vi "Add Subscriber.vi"(8 "error in (no error)":errorcluster, 10 "New FIFO Instance Config":T2 {"Custom Data" format="%.0x"}, 11 "CIF_CIPC_Chn in":refnum<class "CIF_CIPC_Chn.lvclass">) -> (0 "error out":errorcluster, 2 "New FIFO Instance":T1 {"Custom Data" format="%.0x"}, 3 "CIF_CIPC_Chn out":refnum<class "CIF_CIPC_Chn.lvclass">)   [LabVIEW 2021, in "CIF_CIPC_Chn.lvclass"]
uses:
  CIF_CIPC_Chn.lvclass
  D:/dev/Packages/CIF_Channels_Core/src/CIFChannels/CIFChannels.lvclass
  ChannelCommon/typedef/New FIFO Instance Configuration.ctl
  ChannelCommon/typedef/New FIFO Instance Response.ctl
  CIFChannels/CIFChannels.lvclass/CIFChannels.ctl
  CIF_CIPC_Chn.lvclass/CIF_CIPC_Chn.ctl
  ChannelCommon/typedef/Errors.ctl
  CIFChannels/Accessors/Read Name.vi
  <vilib>/CIF Foundation/CIF Utilities/Errors/Append Error Location.vi
  SubVIs/Flatten Buffer Configuration.vi
  <vilib>/CIF Foundation/CIF CIPC/Utilities/Get Size.vi
  ChannelCommon/Utilities/Unflatten FIFO Config.vi
  ChannelCommon/Utilities/Flatten FIFO Config.vi
  CIFChannels/Accessors/Read Channel State.vi
  CIFChannels/Accessors/Read Custom Config Data.vi
  <vilib>/CIF Foundation/CIF Utilities/DataTypes/Flatten Unflatten/Flatten U32.vi
  <vilib>/CIF Foundation/CIF Utilities/DataTypes/Flatten Unflatten/Flatten I32.vi
  <vilib>/CIF Foundation/CIF Utilities/DataTypes/Flatten Unflatten/Flatten U64.vi
  <vilib>/CIF Foundation/CIF CIPC/SubVIs/Check Error.vi
  <vilib>/CIF Foundation/CIF CIPC/SubVIs/Get dll Path.vi
  <vilib>/CIF Foundation/CIF Utilities/DataTypes/Flatten Unflatten/Unflatten U64.vi
  <vilib>/Utility/error.llb/Trim Whitespace.vi
  <vilib>/Utility/error.llb/Error Cluster From Error Code.vi
  ChannelCommon/ChannelCommon.lvlib
  CIFChannels/CIFChannels.lvclass
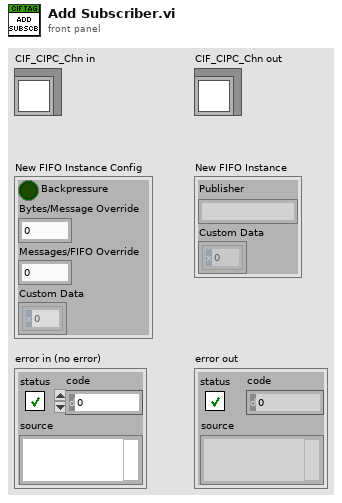
[diagram p1: front panel]
types:
  T1 = typedef "ChannelCommon.lvlib/New FIFO Instance Response.ctl" = cluster{"Publisher":string, "Custom Data":u8[]}
  T2 = typedef "ChannelCommon.lvlib/New FIFO Instance Configuration.ctl" = cluster{"Backpressure":bool, "Bytes/Message Override":u32, "Messages/FIFO Override":u32, "Custom Data":u8[]}
  T3 = typedef "ChannelCommon.lvlib/Errors.ctl" = enum16{"gRPC Server Not Found", "Duplicate Channel", "Missing Channel", "Incorrect Type", "Flatten Error", "Unflatten Data", "Channel Length", "Plugin Connection", "gRPC Server Connection", "FIFO Unflatten", "Required Override", "Remove Not Found", "Multi Sub Not Supported", "Primary Already Connected", "Backpressure Not Supported", "Unable to Increase Buffer"}
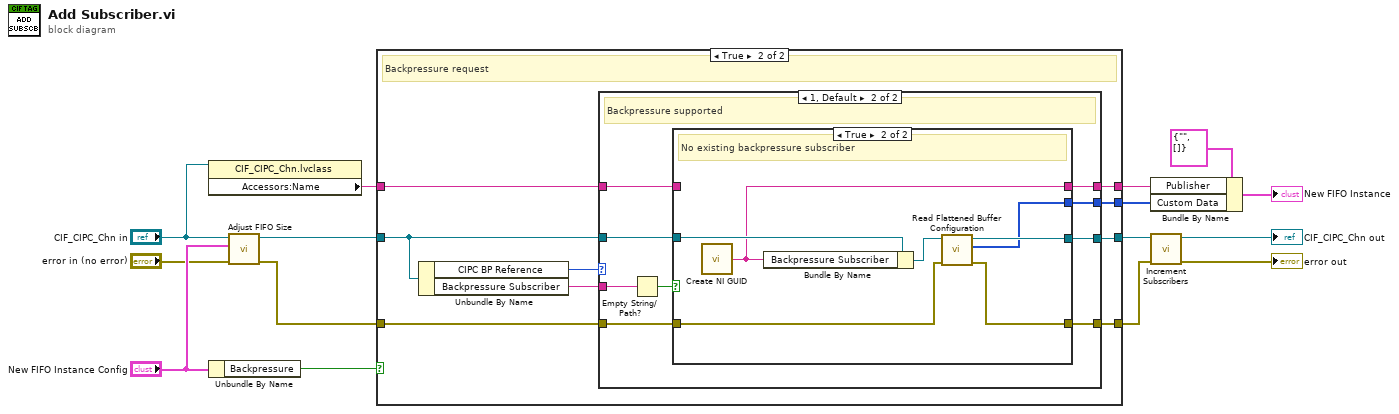
[diagram p0: block diagram]
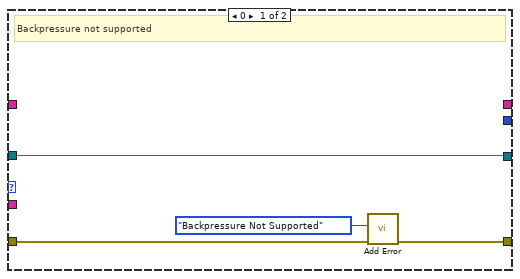
[diagram p3: hidden frame]
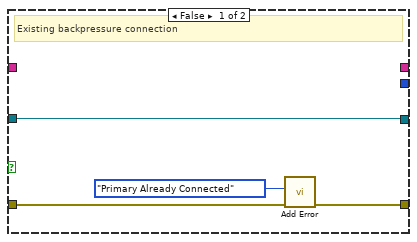
[diagram p4: hidden frame]
diagram:
  n1 = property class="CIF_CIPC_Chn.lvclass"(reference="CIF_CIPC_Chn in") -> ("Accessors:Name"=w14:string)  [unwired: 1 in, 2 out]
  n2 = Unbundle By Name("New FIFO Instance Config") -> ("Backpressure"=w15:bool)
  n3 = call "Adjust FIFO Size.vi"("error in (no error)"="error in (no error)", "New FIFO Instance Config"="New FIFO Instance Config", "CIF_CIPC_Chn in"="CIF_CIPC_Chn in") -> ("error out"=w6:errorcluster, "CIF_CIPC_Chn out"=w9:refnum<class "CIF_CIPC_Chn.lvclass">)  [unwired: 7 in]
  n4 = case shown="True" w15 {
    tunnel: w6 -> [w18 w24]
    tunnel: w14 -> [w16 w23]
    tunnel: w9 -> [w17 w25]
    tunnel: [w16 w22] -> w12
    tunnel: [w18 w21] -> w4
    tunnel: [w17 w20] -> w5
    tunnel: [_ w19] -> w1
    frame False {
      # "No backpressure request"
    }
    frame True {
      # "Backpressure request"
      n5 = Unbundle By Name(w25) -> ("CIPC BP Reference"=w27:u64, "Backpressure Subscriber"=w26:string)
      n6 = case shown="1, Default" w27 {
        tunnel: w26 -> [_ w33]
        tunnel: w25 -> [w31 w40]
        tunnel: w24 -> [w29 w39]
        tunnel: w23 -> [_ w38]
        tunnel: [_ w37] -> w22
        tunnel: [w28 w36] -> w21
        tunnel: [w31 w35] -> w20
        tunnel: [_ w34] -> w19
        frame 0 {
          # "Backpressure not supported"
          n7 = call "Add Error.vi"("error in (no error)"=w29, "Error"=Errors."Backpressure Not Supported") -> ("error out"=w28:errorcluster)  [unwired: 9 in]
        }
        frame 1, Default {
          # "Backpressure supported"
          n8 = Empty String/Path?(string/path=w33) -> (empty?=w32:bool)
          n9 = case shown="True" w32 {
            tunnel: w40 -> [w44 w51]
            tunnel: w39 -> [w42 w49]
            tunnel: w38 -> [_ _]
            tunnel: [_ w46] -> w37
            tunnel: [w41 w48] -> w36
            tunnel: [w44 w47] -> w35
            tunnel: [_ w45] -> w34
            frame False {
              # "Existing backpressure connection"
              n10 = call "Add Error.vi"("error in (no error)"=w42, "Error"=Errors."Primary Already Connected") -> ("error out"=w41:errorcluster)  [unwired: 9 in]
            }
            frame True {
              # "No existing backpressure subscriber"
              n11 = call <vilib>:"Create NI GUID.vi"() -> ("NI GUID"=w46:string)
              n12 = Bundle By Name(cluster=w51, "Backpressure Subscriber"=w46) -> (w50:refnum<class "CIF_CIPC_Chn.lvclass">)
              n13 = call "Read Flattened Buffer Configuration.vi"("error in (no error)"=w49, "CIF_CIPC_Chn in"=w50) -> ("error out"=w48:errorcluster, "Flattened Configuration"=w45:u8[], "CIF_CIPC_Chn out"=w47:refnum<class "CIF_CIPC_Chn.lvclass">)  [unwired: 7 in]
            }
          }
        }
      }
    }
  }
  n14 = Bundle By Name(cluster=T1 {"Publisher"="", "Custom Data"=[]} ("New FIFO Instance"), "Publisher"=w12, "Custom Data"=w1) -> (→"New FIFO Instance":T1)
  n15 = call "Increment Subscribers.vi"("error in (no error)"=w4, "CIFChannels in"=w5) -> ("error out"=→"error out":errorcluster, "CIFChannels out"=→"CIF_CIPC_Chn out":refnum<class "CIF_CIPC_Chn.lvclass">)  [unwired: 8 in]
